vi "图像采样.vi"() -> ()   [LabVIEW 2018]
uses:
  <vilib>/vision/NI_Vision_Development_Module.lvlib
panel:
  out "Image 2":T1(plugin-control)
  out "Image":T1(plugin-control)
  in  "路径":path
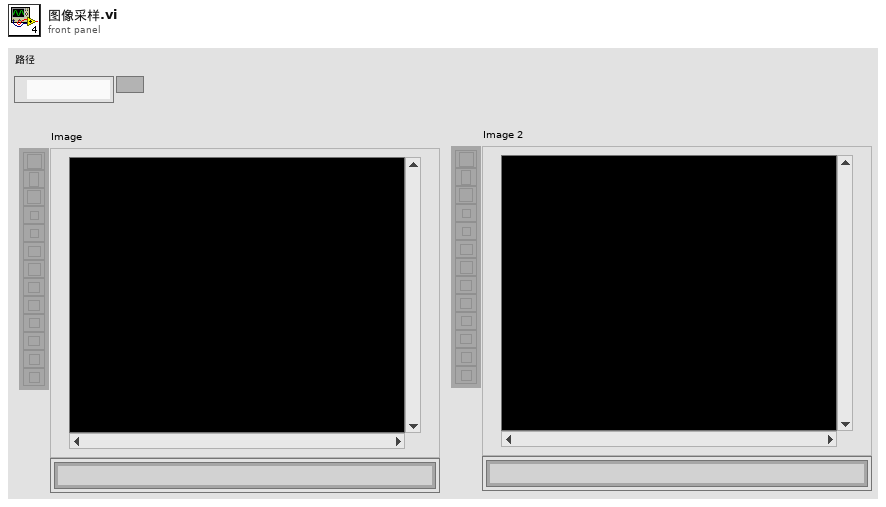
[diagram p1: front panel]
types:
  T1 = typedef "IMAQ Image.ctl" = refnum<image>
  T2 = typedef "Image Type" = u32
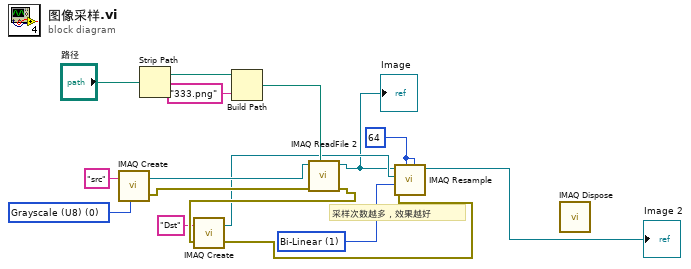
[diagram p0: block diagram]
diagram:
  w7 = u32 1 items=["Zero Order", "Bi-Linear", "Quadratic", "Cubic Spline"] ("Interpolation Type")
  w8 = 64 ("Y Resolution")
  w10 = T2 0 items=["Grayscale (U8)", "Grayscale (I16)", "Grayscale (SGL)", "Complex (CSG)", "RGB (U32)", "HSL (U32)", "RGB (U64)", "Grayscale (U16)"] ("Image Type")
  # "采样次数越多，效果越好"
  n1 = call "IMAQ Create"("Image Name"="src", "Image Type"=w10) -> ("New Image"=w13:T1, "error out"=w12:errorcluster)  [unwired: 3 in]
  n2 = Strip Path(path="路径") -> (stripped path=w15:path)  [unwired: 1 out]
  n3 = Build Path(base path=w15, name or relative path="333.png" ("名称或相对路径")) -> (appended path=w9:path)
  n4 = call "IMAQ ReadFile 2"("File Path"=w9, "error in (no error)"=w12, "Image"=w13) -> ("error out"=w6:errorcluster, "Image Out"=w3:T1)  [unwired: 4 in, 3 out]
  "Image" <- w3
  n5 = call "IMAQ Create"("Image Name"="Dst", "error in (no error)"=w6) -> ("New Image"=w4:T1, "error out"=w5:errorcluster)  [unwired: 3 in]
  n6 = call "IMAQ Resample"("X Resolution"=w8, "Y Resolution"=w8, "error in (no error)"=w5, "Interpolation Type"=w7, "Image Dst"=w4, "Image Src"=w3) -> ("Image Dst Out"=→"Image 2":T1)  [unwired: 4 in, 1 out]
  n7 = call "IMAQ Dispose"() -> ()  [unwired: 6 in, 1 out]
